vi "DSA Measure Signal Amplitude and Levels.vi"(0 "AI Task ID In":refnum<k21>, 1 "AO Task ID In":refnum<k21>[](array[refnum]), 3 "Step Delay Time has Elapsed":bool, 4 "Test Time has Elapsed":bool, 5 "error in":errorcluster, 7 "samples per channel":i32=-1, 11 "Run Mode (Manual = True)":bool) -> (10 "Load Data":bool, 14 "Task ID Cluster":T1, 15 "DSA Measurements Array":sgl[][](array[numeric]), 16 "DSA Measurements":T3, 17 "DSA Functions":T2, 18 "Temperature Data":sgl[](array[numeric]), 19 "error out":errorcluster)   [LabVIEW 2021]
uses:
  Controls/DSA Measurements.ctl
  Controls/DSA Readings.ctl
  Controls/DSA Functions.ctl
  <vilib>/DAQmx/read.llb/DAQmx Read (Analog 1D DBL NChan 1Samp).vi
  <vilib>/DAQmx/read.llb/DAQmx Read (Analog 1D Wfm NChan NSamp).vi
  <vilib>/DAQmx/create/channels.llb/DAQmx Create Channel (AI-Temperature-Thermocouple).vi
  <vilib>/DAQmx/configure/timing.llb/DAQmx Timing (Sample Clock).vi
  <vilib>/DAQmx/miscellaneous.llb/DAQmx Fill In Error Info.vi
  <vilib>/measure/madcrms.llb/Basic Averaged DC-RMS for N Chan.vi
  <vilib>/measure/NI_MAPro.lvlib
  <resource>/objmgr/daqmx.rc
panel:
  in  "Timeout":dbl=10.0 format="%0.2f"
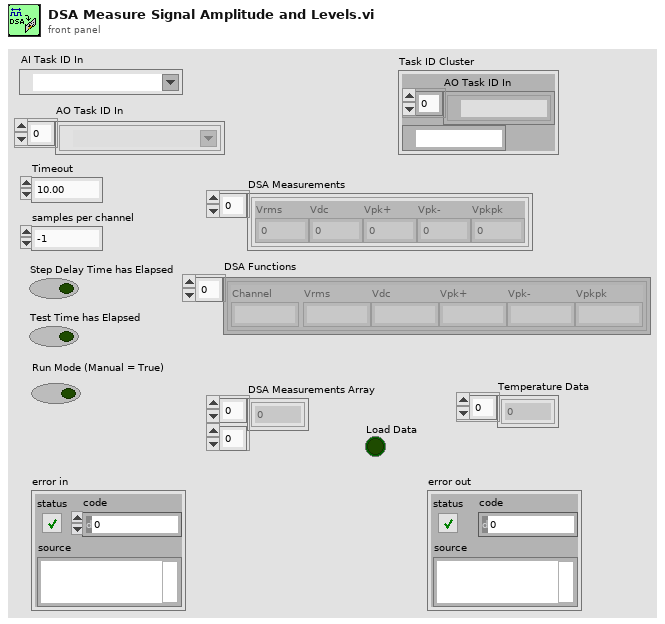
[diagram p1: front panel]
types:
  T1 = cluster{"AO Task ID In":refnum<k21>[], "task out":refnum<k21>}
  T2 = typedef "DSA Functions.ctl" = cluster{"Channel":string, "Vrms":string, "Vdc":string, "Vpk+":string, "Vpk-":string, "Vpkpk":string}[]
  T3 = typedef "DSA Measurements.ctl" = T4[]
  T4 = typedef "DSA Readings.ctl" = cluster{"Vrms":sgl, "Vdc":sgl, "Vpk+":sgl, "Vpk-":sgl, "Vpkpk":sgl}
  T5 = cluster{"[0]":string, "[1]":string, "[2]":string, "[3]":string, "[4]":string, "[5]":string}[]
  T6 = cluster{"Numeric":dbl, "Numeric":dbl, "-Peak value":dbl, "+Peak value":dbl, "Peak-Peak value":dbl}[]
  T7 = enum16{"Rectangular (none)", "Hanning", "Low side lobe"}
  T8 = cluster{"[0]":string, "[1]":string, "[2]":string, "[3]":string, "[4]":string, "[5]":string}
  T9 = cluster{dbl, "Numeric":dbl, "-Peak value":dbl, "+Peak value":dbl, "Peak-Peak value":dbl}
  T10 = cluster{"Numeric":dbl, "Numeric":dbl, "-Peak value":dbl, "+Peak value":dbl, "Peak-Peak value":dbl}
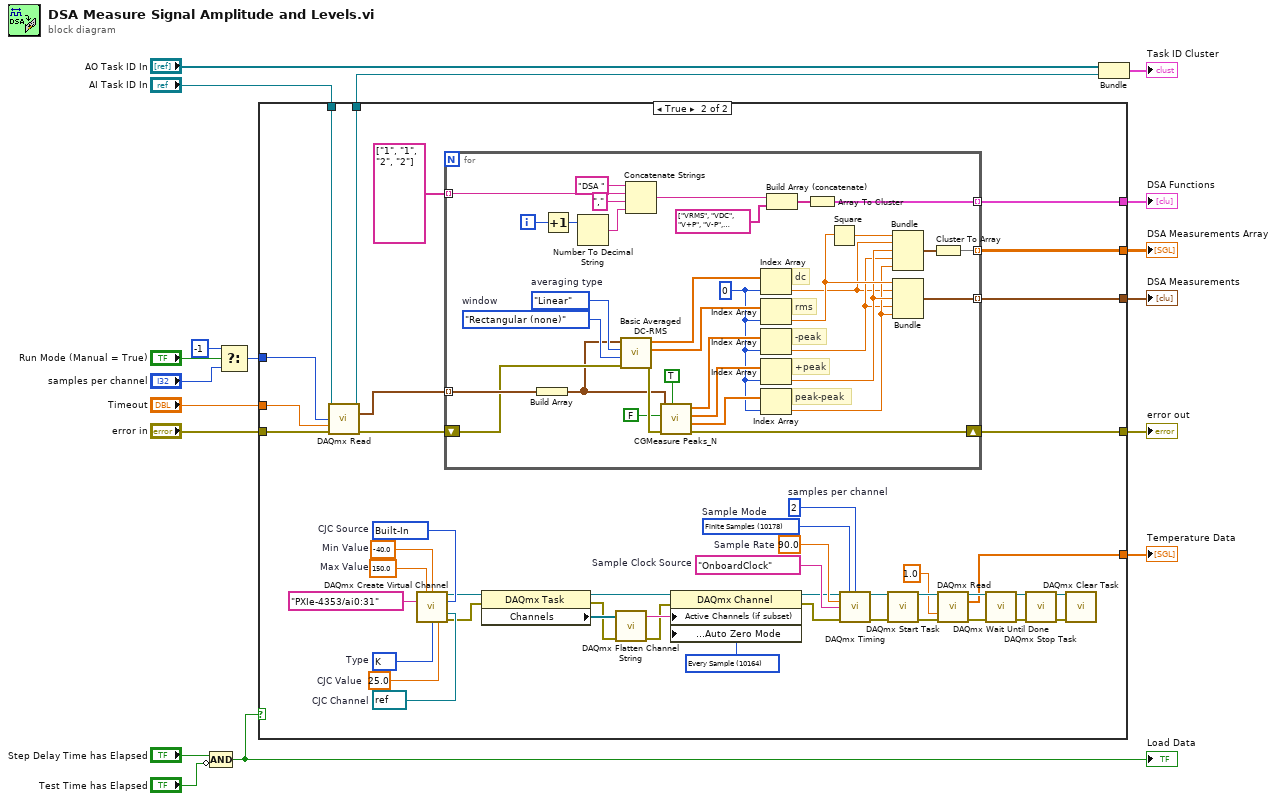
[diagram p0: block diagram]
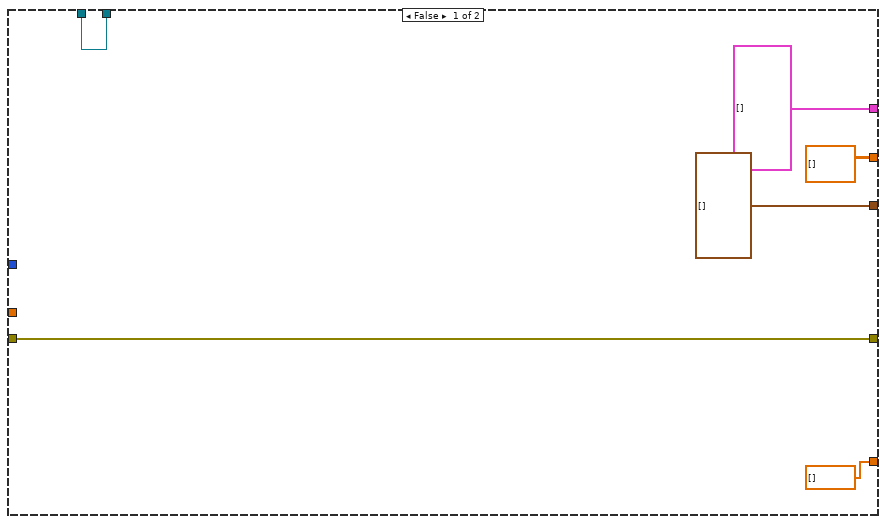
[diagram p2: hidden frame]
diagram:
  n1 = Compound Arithmetic op=AND("Step Delay Time has Elapsed", invert "Test Time has Elapsed") -> (w11:bool)
  "Load Data" <- w11
  n2 = Select(t=-1, s="Run Mode (Manual = True)", f="samples per channel") -> (s? t:f=w2:i32)
  n3 = case shown="True" w11 {
    tunnel: [T6 [] w69] -> w18
    tunnel: "Timeout" -> [_ w68]
    tunnel: [dbl[][] [] w67] -> w16
    tunnel: "error in" -> [w23 w66]
    tunnel: "AI Task ID In" -> [w24 w65]
    tunnel: [w23 w64] -> w6
    tunnel: [T5 [] w63] -> w15
    tunnel: [w24 w62] -> w7
    tunnel: w2 -> [_ w30]
    tunnel: [dbl[] [] ("data") w25] -> w1
    frame False {
    }
    frame True {
      w31 = 2  # samples per channel
      w37 = 10164 items=["None"=10230, "Once"=10244, "Every Sample"=10164] ("Auto Zero Mode")
      w55 = refnum<k21> refnum  # CJC Channel
      w50 = 10200 items=["Built-In"=10200, "Constant Value"=10116, "Channel"=10113]  # CJC Source
      w51 = -40.0  # Min Value
      w52 = 150.0  # Max Value
      w54 = 25.0  # CJC Value
      w53 = 10073 items=["J"=10072, "K"=10073, "N"=10077, "R"=10082, "S"=10085, "T"=10086, "B"=10047, "E"=10055]  # Type
      w47 = 90.0  # Sample Rate
      w48 = tag "OnboardClock"  # Sample Clock Source
      w49 = 10178 items=["Finite Samples"=10178, "Continuous Samples"=10123, "Hardware Timed Single Point"=12522]  # Sample Mode
      n4 = call-poly <vilib>:"DAQmx Read.vi"("task/channels in"=w65, "number of samples per channel"=w30, "timeout"=w68, "error in"=w66) -> ("task out"=w62:refnum<k21>, "data"=w61:waveform(dbl)[], "error out"=w60:errorcluster)  [unwired: 9 in]
      n5 = call-poly <vilib>:"DAQmx Create Virtual Channel.vi"("maximum value"=w52, "minimum value"=w51, "physical channels"=tag "PXIe-4353/ai0:31" ("Physical Channel"), "cjc source"=w50, "cjc channel"=w55, "thermocouple type"=w53, "cjc value"=w54) -> ("task out"=w46:refnum<k21>, "error out"=w44:errorcluster)  [unwired: 7 in]
      n6 = for {
        tunnel: w61 -> [w103] mode=indexing
        shift-right: [w101] -> w64
        shift-left: w60 -> [w102]
        tunnel: [w90] -> w67 mode=indexing
        tunnel: [w89] -> w69 mode=indexing
        tunnel: [w79] -> w63 mode=indexing
        tunnel: string[] ["1", "1", "2", "2"] ("Array") -> [w78] mode=indexing
        i -> [w80]
        w88 = 0 ("index")
        w98 = T7."Rectangular (none)"  # window
        w99 = enum16{"Linear", "Exponential"}."Linear"  # averaging type
        # "+peak"
        # "peak-peak"
        # "-peak"
        # "rms"
        # "dc"
        n7 = Build Array(w103) -> (w87:waveform(dbl)[])
        n8 = Increment(x=w80) -> (x+1=w83:i32)
        n9 = Number To Decimal String(number=w83) -> (decimal integer string=w84:string)  [unwired: 1 in]
        n10 = call-poly <vilib>:"Basic Averaged DC-RMS.vi"("error in (no error)"=w102, "window"=w98, "averaging type"=w99, "signals in"=w87) -> ("error out"=w100:errorcluster, "RMS values"=w95:dbl[], "DC values"=w96:dbl[])  [unwired: 4 in, 1 out]
        n11 = Concatenate Strings("DSA " ("string"), w78, "," ("string"), w84) -> (w85:string)
        n12 = call <vilib>:"CGMeasure Peaks_N.vi"("reset"=TRUE, "error in (no error)"=w100, "hold"=FALSE ("hold peaks"), "signals in"=w87) -> ("error out"=w101:errorcluster, "Peak-Peak values"=w92:dbl[], "-Peak values"=w93:dbl[], "+Peak values"=w94:dbl[])  [unwired: 4 in]
        n13 = Index Array(array=w96, index=w88) -> (element=w72:dbl)
        n14 = Index Array(array=w95, index=w88) -> (element=w76:dbl)
        n15 = Index Array(array=w94, index=w88) -> (element=w73:dbl)
        n16 = Index Array(array=w93, index=w88) -> (element=w75:dbl)
        n17 = Index Array(array=w92, index=w88) -> (element=w74:dbl)
        n18 = Build Array (concatenate)(w85, string[] ["VRMS", "VDC", "V+P", "V-P", "VPkPk"] ("DSA Functions")) -> (w86:string[])
        n19 = Array To Cluster(array=w86) -> (cluster=w79:T8)
        n20 = Square(x=w76) -> (x^2=w70:dbl)
        n21 = Bundle(w70, "Numeric"=w72, "-Peak value"=w75, "+Peak value"=w73, "Peak-Peak value"=w74) -> (w71:T9)  [unwired: 1 in]
        n22 = Bundle("Numeric"=w76, "Numeric"=w72, "-Peak value"=w75, "+Peak value"=w73, "Peak-Peak value"=w74) -> (w89:T10)  [unwired: 1 in]
        n23 = Cluster To Array(cluster=w71) -> (array=w90:dbl[])
      }
      n24 = property class="DAQmx Task"(reference=w46, error in=w44) -> (reference out=w42:refnum<k21>, error out=w39:errorcluster, "Channels"=w41:refnum<k21>[])
      n25 = call <vilib>:"DAQmx Flatten Channel String.vi"("names in"=w41, "error in"=w39) -> ("names out"=w40:string, "error out"=w38:errorcluster)  [unwired: 12 in]
      n26 = property class="DAQmx Channel"(reference=w42, error in=w38, "Active Channels (if subset)"=w40, "Analog Input:General Properties:Advanced:High Accuracy Settings:Auto Zero Mode"=w37) -> (reference out=w45:refnum<k21>, error out=w43:errorcluster)
      n27 = call-poly <vilib>:"DAQmx Timing.vi"("task/channels in"=w45, "sample mode"=w49, "samples per channel"=w31, "rate"=w47, "source"=w48, "error in"=w43) -> ("task out"=w56:refnum<k21>, "error out"=w36:errorcluster)  [unwired: 8 in]
      n28 = call <vilib>:"DAQmx Start Task.vi"("task/channels in"=w56, "error in"=w36) -> ("task out"=w34:refnum<k21>, "error out"=w33:errorcluster)  [unwired: 12 in]
      n29 = call-poly <vilib>:"DAQmx Read.vi"("task/channels in"=w34, "timeout"=1.0, "error in"=w33) -> ("task out"=w29:refnum<k21>, "data"=w25:dbl[], "error out"=w27:errorcluster)  [unwired: 10 in]
      n30 = call <vilib>:"DAQmx Wait Until Done.vi"("task/channels in"=w29, "error in"=w27) -> ("task out"=w28:refnum<k21>, "error out"=w26:errorcluster)  [unwired: 12 in]
      n31 = call <vilib>:"DAQmx Stop Task.vi"("task/channels in"=w28, "error in"=w26) -> ("task out"=w58:refnum<k21>, "error out"=w57:errorcluster)  [unwired: 12 in]
      n32 = call <vilib>:"DAQmx Clear Task.vi"("task in"=w58, "error in"=w57) -> ()  [unwired: 13 in, 1 out]
    }
  }
  "DSA Measurements" <- w18
  "DSA Measurements Array" <- w16
  "DSA Functions" <- w15
  "error out" <- w6
  "Temperature Data" <- w1
  n33 = Bundle("AO Task ID In"="AO Task ID In", "task out"=w7) -> (→"Task ID Cluster":T1)  [unwired: 1 in]
